vi "CreateNotification.vi"(11 "name":string="print") -> (3 "notification":string)   [LabVIEW 2011]
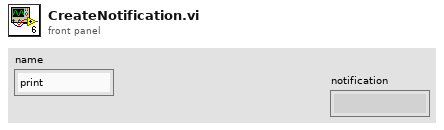
[diagram p1: front panel]
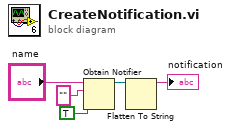
[diagram p0: block diagram]
diagram:
  n1 = Obtain Notifier(name (unnamed)="name", notification data type="" ("名称（未命名）"), create if not found? (T)=TRUE ("如未找到是否创建？(T)")) -> (notifier out=w3:refnum<notifier>)  [unwired: 1 in, 2 out]
  n2 = Flatten To String(anything=w3) -> (data string=→"notification":string)  [unwired: 3 in, 2 out]
